vi "Test Open Send.vi"() -> ()   [LabVIEW 2016, in "RemoteControl.STM.lvclass"]
uses:
  RemoteControl.STM/RemoteControl.STM.lvclass
  Typedefs/Message--Cluster.ctl
  RemoteControl.v2.lvclass
panel:
  out "error out":errorcluster
  in  "Message":T1
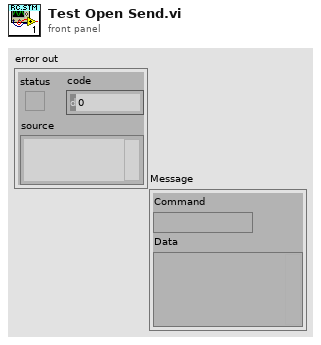
[diagram p1: front panel]
types:
  T1 = typedef "RemoteControl.v2.lvclass/Message--Cluster.ctl" = cluster{"Command":string, "Data":variant}
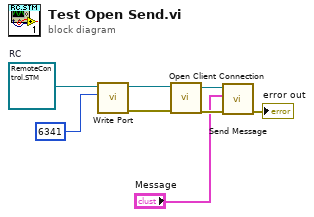
[diagram p0: block diagram]
diagram:
  w6 = refnum<class "RemoteControl.STM.lvclass"> refnum  # RC
  n1 = call-dynamic "Write Port.vi"("Port"=u32 6341, "RemoteControl in"=w6) -> ("error out"=w7:errorcluster, "RemoteControl out"=w8:refnum<class "RemoteControl.STM.lvclass">)  [unwired: 8 in]
  n2 = call-dynamic "Open Client Connection.vi"("error in (no error)"=w7, "RemoteControl.STM in"=w8) -> ("error out"=w4:errorcluster, "RemoteControl.STM out"=w5:refnum<class "RemoteControl.STM.lvclass">)  [unwired: 8 in]
  n3 = call-dynamic "Send Message.vi"("error in (no error)"=w4, "Message"="Message", "RemoteControl.STM in"=w5) -> ("error out"=→"error out":errorcluster)  [unwired: 7 in, 1 out]
